vi "Render Non-False Value Section.vi"(8 "Error In":errorcluster) -> (0 "Error Out":errorcluster)   [LabVIEW 2018, in "Tests.lvlib" / "Render.lvlib"]
uses:
  Render.lvlib
  src/Toolkit/Data/Map/Map.lvclass
  D:/Users/cfield/Code/Field R&D Services/Mustache/trunk/src/Toolkit/Data/Abstract/Abstract.lvclass
  src/Toolkit/Low-Level/Support/Lex String.vi
  src/Toolkit/Data/Map/Support/From String.vi
  src/Toolkit/Data/Map/Support/From Datum.vi
  src/Toolkit/Low-Level/Support/Render to String.vi
  <vilib>/addons/_JKI Toolkits/Caraya/classes/Test/Test.lvclass
  <vilib>/addons/_JKI Toolkits/Caraya/classes/Assert/Assert.lvclass
  src/Toolkit/Toolkit.lvlib
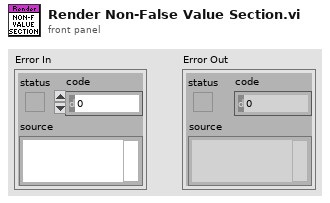
[diagram p1: front panel]
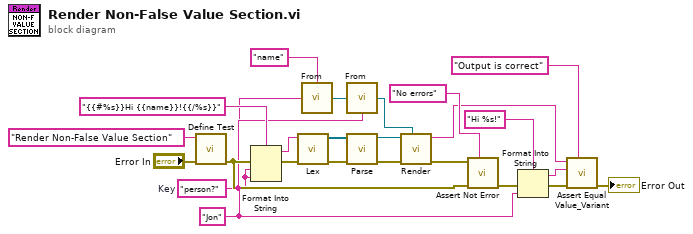
[diagram p0: block diagram]
diagram:
  w1 = "Jon" ("Value")
  w8 = "person?"  # Key
  n1 = call <vilib>:"Define Test.vi"("error in (no error)"="Error In", "Label (VI Title)"="Render Non-False Value Section") -> ("error out"=w12:errorcluster)  [unwired: 9 in]
  n2 = Format Into String(format string="{{#%s}}Hi {{name}}!{{/%s}}", error in=w12, w8, w8) -> (resulting string=w9:string, error out=w11:errorcluster)  [unwired: 1 in]
  n3 = call-poly "Lex.vi"("Error In"=w11, "Input"=w9) -> ("Error Out"=w14:errorcluster, "Tokens"=w15:refnum<class "Abstract.lvclass">[])  [unwired: 8 in]
  n4 = call-poly "From.vi"("Value"=w1, "Key"="name") -> ("Map"=w6:refnum<class "Map.lvclass">)
  n5 = call-poly "From.vi"("Value"=w6, "Key"=w8) -> ("Map"=w13:refnum<class "Map.lvclass">)
  n6 = call "Parse.vi"("Error In"=w14, "Tokens"=w15) -> ("Error Out"=w16:errorcluster, "Abstract Syntax Tree"=w7:refnum<class "Root.lvclass">)  [unwired: 8 in]
  n7 = call-poly "Render.vi"("Data"=w13, "Error In"=w16, "Abstract Syntax Tree"=w7) -> ("Error Out"=w18:errorcluster, "Output"=w17:string)  [unwired: 7 in]
  n8 = call <vilib>:"Assert Not Error.vi"("Label"="No errors", "error in (no error)"=w12, "Not Error?"=w18) -> ("error out"=w21:errorcluster)  [unwired: 8 in]
  n9 = Format Into String(format string="Hi %s!", error in=w21, w1) -> (resulting string=w2:string, error out=w4:errorcluster)  [unwired: 1 in]
  n10 = call <vilib>:"Assert Equal Value_Variant.vi"("Label"="Output is correct", "error in (no error)"=w4, "Y"=w2, "X"=w17) -> ("error out"=→"Error Out":errorcluster)  [unwired: 7 in]
